vi "setUp.vi"(8 "error in":errorcluster, 11 "reference in":refnum<class "Single Board 1Ch Loopback.lvclass">) -> (0 "error out":errorcluster, 3 "reference out":refnum<class "Single Board 1Ch Loopback.lvclass">)   [LabVIEW 2020, in "Single Board 1Ch Loopback.lvclass"]
doc: "setUp runs prior to the test method during test execution. Use this method to initialize any object data required by your tests."
uses:
  Single Board 1Ch Loopback.lvclass
  C:/Program Files (x86)/National Instruments/LabVIEW 2020/vi.lib/addons/_JKI Toolkits/VI Tester/TestCase.llb/TestCase.lvclass
  <vilib>/addons/_JKI Toolkits/VI Tester/TestCase.llb/TestCase.lvclass
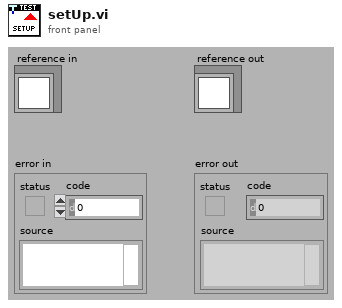
[diagram p1: front panel]
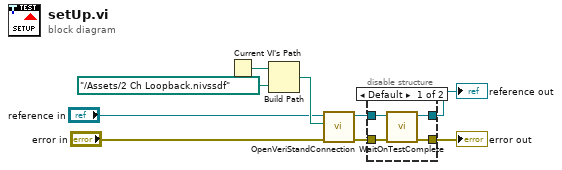
[diagram p0: block diagram]
diagram:
  n1 = Current VI's Path() -> (path=w4:path)
  n2 = Build Path(base path=w4, name or relative path=path "../Assets/2 Ch Loopback.nivssdf") -> (appended path=w3:path)
  n3 = call-dynamic "OpenVeriStandConnection.vi"("error in (no error)"="error in", "System Definition File"=w3, "VeriStand Test Case in"="reference in") -> ("error out"=w7:errorcluster, "VeriStand Test Case out"=w6:refnum<class "Single Board 1Ch Loopback.lvclass">)  [unwired: 6 in, 1 out]
  n4 = disable-structure shown="Default" {
    disable-tunnel: w7 -> [w13 w14]
    disable-tunnel: [w12 w14] -> w9
    disable-tunnel: [w11 w15] -> w8
    disable-tunnel: w6 -> [w10 w15]
    frame condition #0 (active) {
      n5 = call <vilib>:"WaitOnTestComplete.vi"("error in (no error)"=w13, "TestCase in"=w10) -> ("error out"=w12:errorcluster, "TestCase out"=w11:refnum<class "Single Board 1Ch Loopback.lvclass">)  [unwired: 8 in]
    }
    frame condition #1 {
    }
  }
  "error out" <- w9
  "reference out" <- w8
